vi "printDaqServer.vi"(8 "error in":errorcluster, 9 "Indent":i32, 10 "TreeRef":refnum<vi>, 11 "baseObject in":refnum<class "IBaseObject.lvclass">) -> (0 "error out":errorcluster, 3 "baseObject out":refnum<class "IBaseObject.lvclass">)   [LabVIEW 2022 SP3, in "openDAQ.lvlib" / "daqUtils.lvlib" / "Tree.lvlib"]
uses:
  Tree.lvlib
  IServer/IServer.lvclass
  ISignal/ISignal.lvclass
  IBaseObject/IBaseObject.lvclass
  IBaseObject/Polymorphic/queryInterface/queryServerInterface.vi
  IComponent/IComponent.lvclass
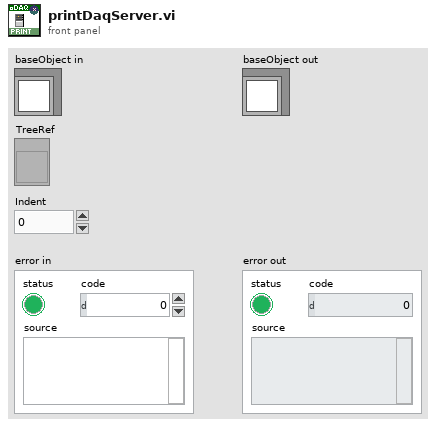
[diagram p1: front panel]
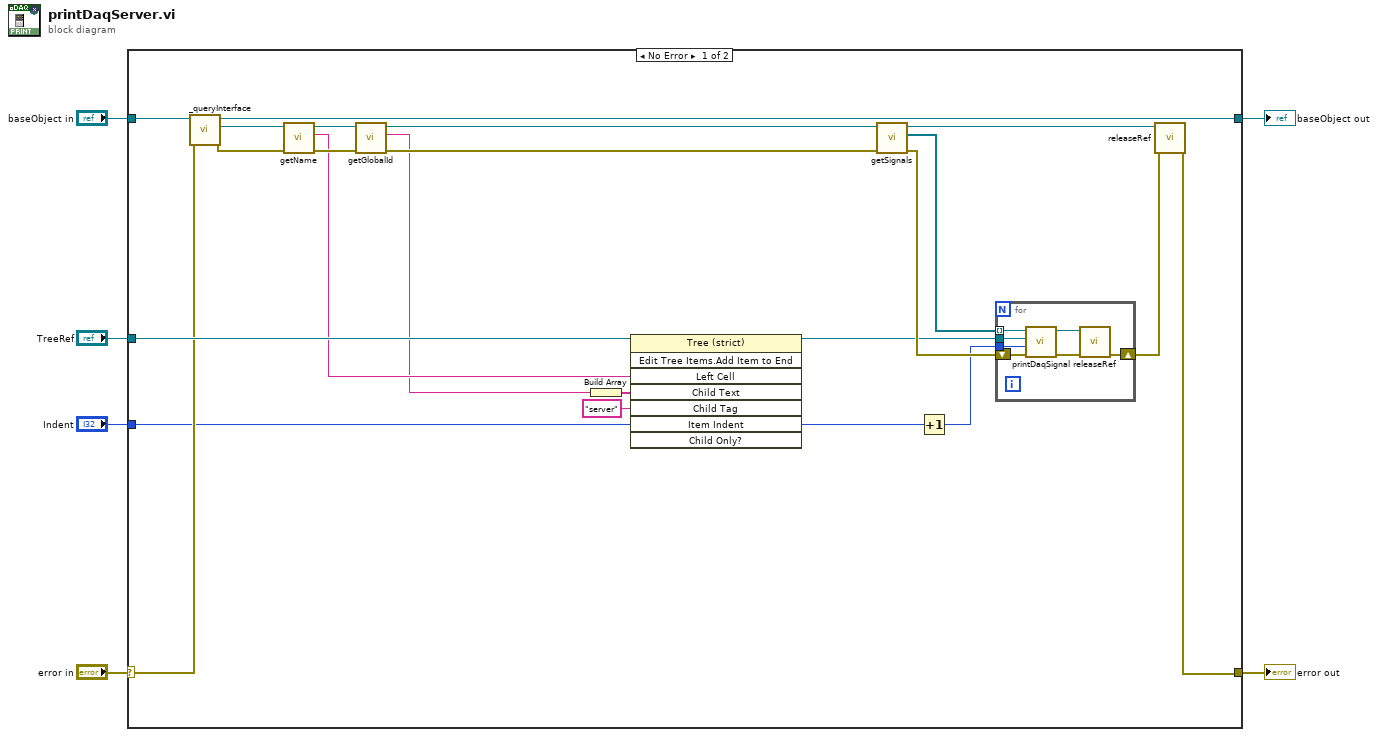
[diagram p0: block diagram]
diagram:
  n1 = case shown="No Error" "error in" {
    selector: "error in" -> [w23 w36]
    tunnel: "baseObject in" -> [w28 w35]
    tunnel: "Indent" -> [w16 _]
    tunnel: "TreeRef" -> [w24 _]
    tunnel: [w22 w36] -> w2
    tunnel: [w26 w35] -> w1
    frame No Error {
      n2 = call-poly "_queryInterface.vi"("error in (no error)"=w23, "IBaseObject in"=w28) -> ("error out"=w25:errorcluster, "IServer out"=w27:refnum<class "IServer.lvclass">, "IBaseObject out"=w26:refnum<class "IBaseObject.lvclass">)  [unwired: 7 in]
      n3 = call "getName.vi"("error in (no error)"=w25, "IComponent in"=w27) -> ("error out"=w12:errorcluster, "Name out"=w9:string, "IComponent out"=w13:refnum<class "IServer.lvclass">)  [unwired: 7 in]
      n4 = call "getGlobalId.vi"("error in (no error)"=w12, "IComponent in"=w13) -> ("error out"=w10:errorcluster, "GlobalId out"=w8:string, "IComponent out"=w11:refnum<class "IServer.lvclass">)  [unwired: 7 in]
      n5 = Build Array(w8) -> (w7:string[])
      n6 = invoke class="Tree (strict)" method="Edit Tree Items.Add Item to End"(reference=w24, "Left Cell"=w9, "Child Text"=w7, "Child Tag"="server", "Item Indent"=w16) -> (reference out=w17:refnum<vi>)  [unwired: 3 in, 7 out]
      n7 = call "getSignals.vi"("error in (no error)"=w10, "IServer in"=w11) -> ("error out"=w20:errorcluster, "Available Signals out"=w19:refnum<class "ISignal.lvclass">[], "IServer out"=w21:refnum<class "IServer.lvclass">)  [unwired: 7 in]
      n8 = Increment(x=w16) -> (x+1=w15:i32)
      n9 = for {
        tunnel: w19 -> [w32] mode=indexing
        shift-right: [w33] -> w18
        shift-left: w20 -> [w34]
        tunnel: w17 -> [w30]
        tunnel: w15 -> [w29]
        n10 = call "printDaqSignal.vi"("Indent"=w29, "TreeRef"=w30, "baseObject in"=w32) -> ("baseObject out"=w31:refnum<class "ISignal.lvclass">)  [unwired: 7 in, 1 out]
        n11 = call-dynamic "releaseRef.vi"("error in (no error)"=w34, "IBaseObject in"=w31) -> ("error out"=w33:errorcluster)  [unwired: 9 in]
      }
      n12 = call-dynamic "releaseRef.vi"("error in (no error)"=w18, "IBaseObject in"=w21) -> ("error out"=w22:errorcluster)  [unwired: 9 in]
    }
    frame Error {
    }
  }
  "error out" <- w2
  "baseObject out" <- w1
